vi "Read Prepend Result Name.vi"(8 "error in (no error)":errorcluster, 11 "Measurement Interface in":refnum<class "Measurement Interface.lvclass">) -> (0 "error out":errorcluster, 2 "Prepend Result Name":bool, 3 "Measurement Interface out":refnum<class "Measurement Interface.lvclass">)   [LabVIEW 2016, in "Measurement Interface.lvlib" / "Measurement Interface.lvclass"]
uses:
  Measurement Interface.lvclass
  Measurement Interface.lvclass/Measurement Interface.ctl
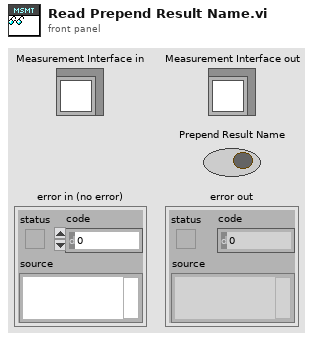
[diagram p1: front panel]
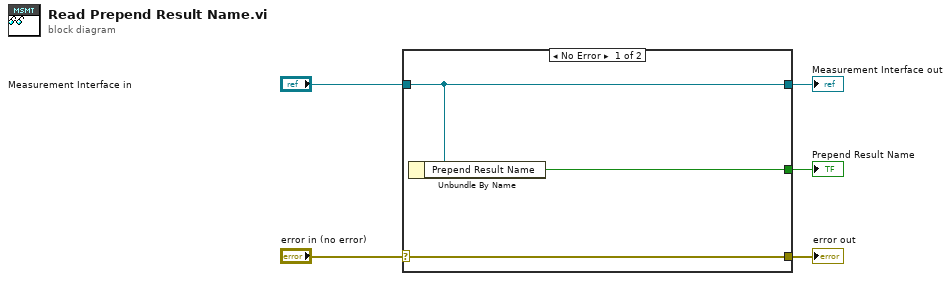
[diagram p0: block diagram]
diagram:
  n1 = case shown="No Error" "error in (no error)" {
    selector: "error in (no error)" -> [w8 w9]
    tunnel: [w8 w9] -> w4
    tunnel: [w7 w10] -> w2
    tunnel: "Measurement Interface in" -> [w7 w10]
    tunnel: [w6 _] -> w1
    frame No Error {
      n2 = Unbundle By Name(w7) -> ("Prepend Result Name"=w6:bool)
    }
    frame Error {
    }
  }
  "error out" <- w4
  "Measurement Interface out" <- w2
  "Prepend Result Name" <- w1
